vi "배열인덱스.vi"() -> ()   [LabVIEW 2014]
panel:
  out "원소":i32
  out "부분배열 2":i32[](array[numeric])
  out "부분배열":i32[](array[numeric])
  out "배열":i32[][](array[numeric])
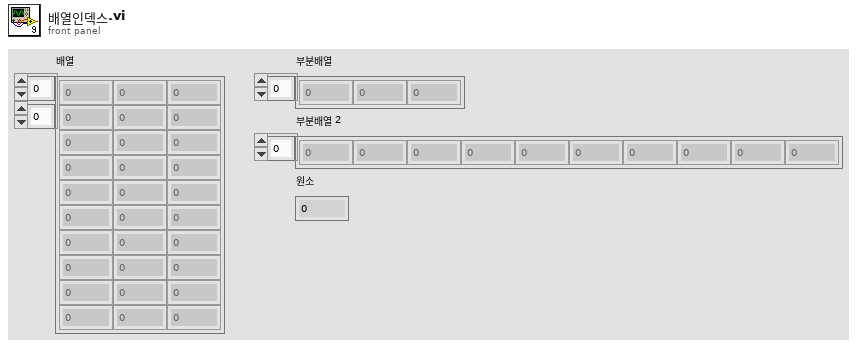
[diagram p1: front panel]
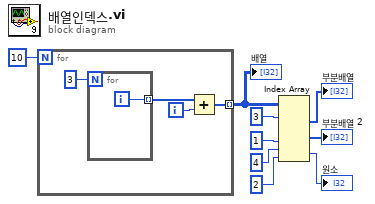
[diagram p0: block diagram]
diagram:
  n1 = for {
    N: 10 -> [_]
    tunnel: [w10] -> w7 mode=indexing
    i -> [w11]
    n2 = for {
      N: 3 -> [_]
      tunnel: [w14] -> w12 mode=indexing
      i -> [w14]
    }
    n3 = Add(x=w12, y=w11) -> (x+y=w10:i32[])
  }
  "배열" <- w7
  n4 = Index Array(array=w7, index (row) #1=3 ("인덱스 (행)"), index (col) #2=1 ("비활성화된 인덱스 (열)"), index (row) #3=4 ("인덱스 (행)"), index (col) #3=2 ("비활성화된 인덱스 (열)")) -> (element #1=→"부분배열":i32[], element #2=→"부분배열 2":i32[], element #3=→"원소":i32)  [unwired: 2 in]
